vi "Carry_Auto.vi"(10 "Carry_Manual":bool, 11 "Ele_At_Pos":bool) -> (2 "Lower to Carry":bool, 3 "Open Arms":bool)   [LabVIEW 2014]
panel:
  in  "Time_Control":i32=50
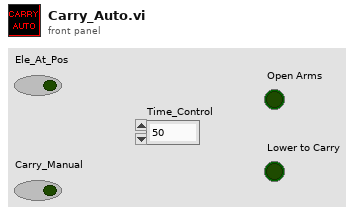
[diagram p1: front panel]
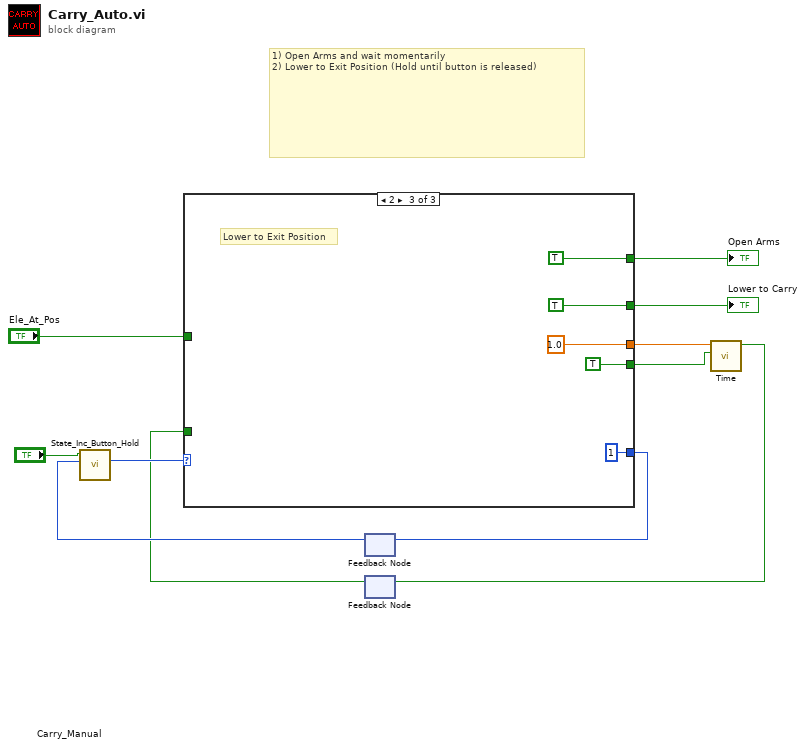
[diagram p0: block diagram]
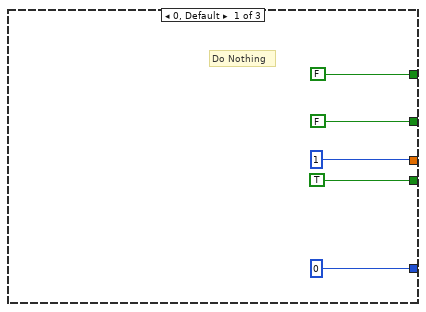
[diagram p2: hidden frame]
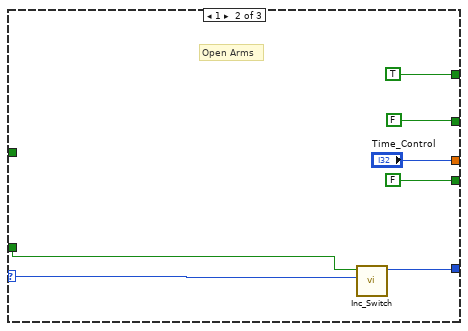
[diagram p3: hidden frame]
diagram:
  # "1) Open Arms and wait momentarily\n2) Lower to Exit Position (Hold until button is released)"
  n1 = feedback #1() -> (w8:i32)  [unwired: 1 in]
  n2 = call "State_Inc_Button_Hold.vi"("Numeric in"=w8, "Floor_Pickup"="Carry_Manual") -> ("t"=w10:i32)  [unwired: 9 in]
  n3 = feedback #2() -> (w1:bool)  [unwired: 1 in]
  n4 = case shown="2" w10 {
    selector: w10 -> [_ w22 _]
    tunnel: [FALSE TRUE TRUE] -> w7
    tunnel: [0 w21 1 ("Numeric out")] -> w11
    tunnel: [FALSE FALSE TRUE] -> w6
    tunnel: "Ele_At_Pos" -> [_ _ _]
    tunnel: [1 "Time_Control" 1.0] -> w3
    tunnel: [TRUE FALSE TRUE] -> w2
    tunnel: w1 -> [_ w17 _]
    frame 0, Default {
      # "Do Nothing"
    }
    frame 1 {
      # "Open Arms"
      n5 = call "Inc_Switch.vi"("Numeric in"=w22, "Ele_At_Pos"=w17) -> ("Numeric out"=w21:i32)  [unwired: 9 in]
    }
    frame 2 {
      # "Lower to Exit Position"
    }
  }
  "Open Arms" <- w7
  "Lower to Carry" <- w6
  n6 = feedback-in #1(w11) -> ()
  n7 = call "Time.vi"("Reset"=w2, "Time_Limit"=w3) -> ("Time_Met"=w4:bool)  [unwired: 9 in]
  n8 = feedback-in #2(w4) -> ()
